vi "LinearSystemId_CreateDriveTrainSystem.vi"(4 "G":dbl, 6 "JKgMetersSquared":dbl, 8 "rbMeters":dbl, 9 "rMeters":dbl, 10 "MassKg":dbl, 11 "Motor":T1 {"Kt_NMPerAmp" format="%13.5p"; "Kv_RadPerSecPerVolt" format="%13.5p"; "R_Ohms" format="%13.5p"; "FreeSpeed_RadPerSec" format="%13.5p"; "FreeCurrent_Amps" format="%13.5p"; "StallCurrent_Amps" format="%13.5p"; "StallTorque_NM" format="%13.5p"; "nominalVoltage_Volts" format="%13.5p"}) -> (3 "Linearsystem":T2)   [LabVIEW 2019, in "Trajectory_Library.lvlib"]
doc: "Creates a new LINEAR SYSTEM data cluster with the specified values. \n\n\nInputs: \n - XXX -- XXX.\n\nOutputs:\n - XXX -- XXX."
uses:
  Trajectory_Library.lvlib
  LINEAR_SYSTEM.ctl
  <vilib>/Analysis/Matrix/Datatypes/RealMatrix.ctl
  DCMOTOR.CTL
  <vilib>/Analysis/Matrix/NI_Matrix.lvlib
panel:
  in  "Outputs":i32=2
  in  "Inputs":i32=2
  in  "States":i32=2
  # "<States,States>"
  # "<States,Inputs>"
  # "<Outputs,States>"
  # "<Outputs,Inputs>"
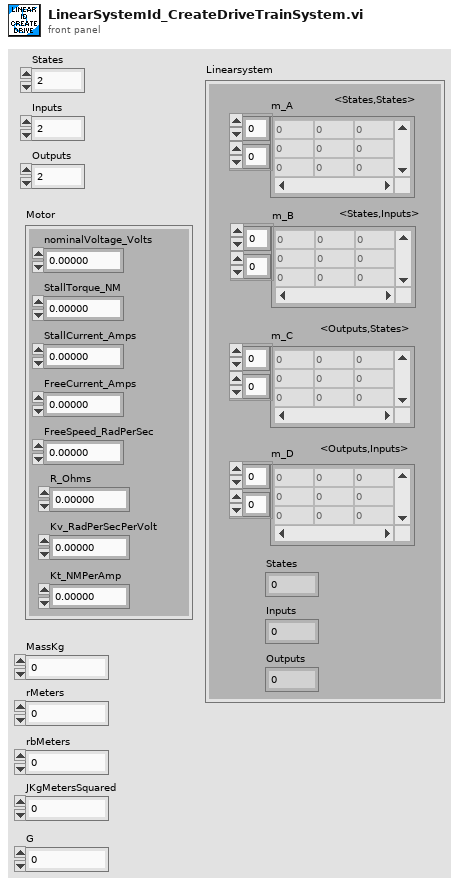
[diagram p1: front panel]
types:
  T1 = typedef "Trajectory_Library.lvlib/DCMOTOR.CTL" = cluster{"nominalVoltage_Volts":dbl, "StallTorque_NM":dbl, "StallCurrent_Amps":dbl, "FreeCurrent_Amps":dbl, "FreeSpeed_RadPerSec":dbl, "R_Ohms":dbl, "Kv_RadPerSecPerVolt":dbl, "Kt_NMPerAmp":dbl}
  T2 = typedef "Trajectory_Library.lvlib/LINEAR_SYSTEM.ctl" = cluster{"m_A":T3, "m_B":T3, "m_C":T3, "m_D":T3, "States":i32, "Inputs":i32, "Outputs":i32}
  T3 = typedef "NI_Matrix.lvlib/RealMatrix.ctl" = dbl[][]
  T4 = typedef "Trajectory_Library.lvlib/LINEARSYSTEM.ctl" = cluster{"m_A":T3, "m_B":T3, "m_C":T3, "m_D":T3, "States":i32, "Inputs":i32, "Outputs":i32}
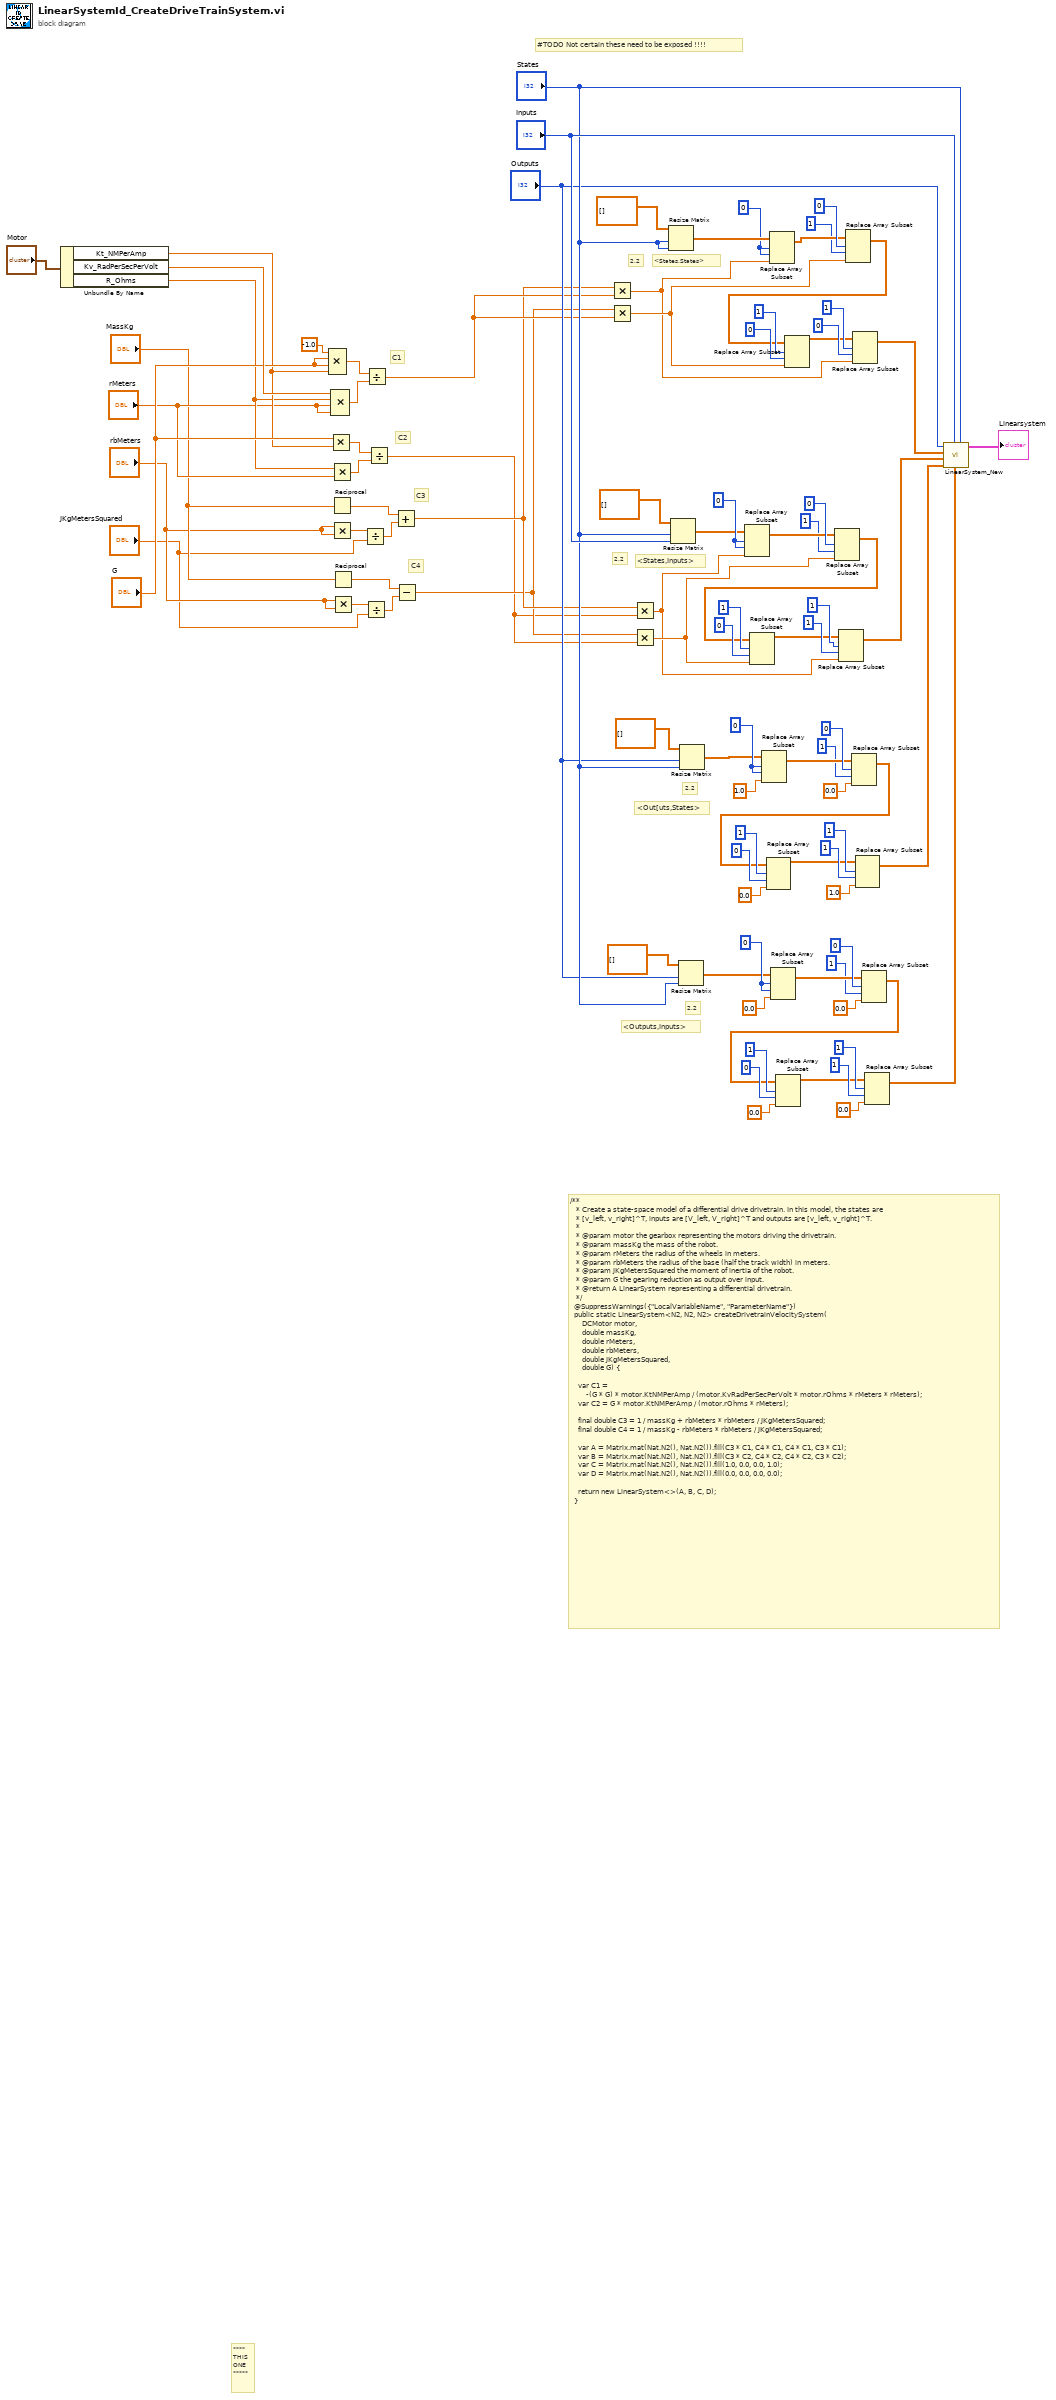
[diagram p0: block diagram]
diagram:
  w40 = 0 ("index (col)")
  w56 = 0 ("index (col)")
  w86 = 0 ("index (col)")
  w89 = 0 ("index (col)")
  # "C4"
  # "C3"
  # "C2"
  # "C1"
  # "2,2"
  # "2,2"
  # "2,2"
  # "2,2"
  # "<States,States>"
  # "<States,Inputs>"
  # "<Out[uts,States>"
  # "<Outputs,Inputs>"
  # "#TODO Not certain these need to be exposed !!!!"
  # "/**\n   * Create a state-space model of a differential drive drivetrain. In this model, the states are\n   * [v_left, v_right]^T, inputs are [V_left, V_right]^T and outputs are [v_left, v_right]^T.\n   *\n   * @param motor the gearbox representing the motors driving the drivetrain.\n   * @param massKg the mass of the robot.\n   * @param rMeters the radius of the wheels in meters.\n   * @param rbMeters the radius of the base (half the track width) in meters.\n   * @param JKgMetersSquared the moment of inertia of the robot.\n   * @param G the gearing reduction as output over input.\n   * @return A LinearSystem representing a differential drivetrain.\n   */\n  @SuppressWarnings({\"LocalVariableName\", \"ParameterName\"})\n  public static LinearSystem<N2, N2, N2> createDrivetrainVelocitySystem(\n      DCMotor motor,\n      double massKg,\n      double rMeters,\n      double rbMeters,\n      double JKgMetersSquared,\n      double G) {\n\n    var C1 =\n        -(G * G) * motor.KtNMPerAmp / (motor.KvRadPerSecPerVolt * motor.rOhms * rMeters * rMeters);\n    var C2 = G * motor.KtNMPerAmp / (motor.rOhms * rMeters);\n\n    final double C3 = 1 / massKg + rbMeters * rbMeters / JKgMetersSquared;\n    final double C4 = 1 / massKg - rbMeters * rbMeters / JKgMetersSquared;\n\n    var A = Matrix.mat(Nat.N2(), Nat.N2()).fill(C3 * C1, C4 * C1, C4 * C1, C3 * C1);\n    var B = Matrix.mat(Nat.N2(), Nat.N2()).fill(C3 * C2, C4 * C2, C4 * C2, C3 * C2);\n    var C = Matrix.mat(Nat.N2(), Nat.N2()).fill(1.0, 0.0, 0.0, 1.0);\n    var D = Matrix.mat(Nat.N2(), Nat.N2()).fill(0.0, 0.0, 0.0, 0.0);\n\n    return new LinearSystem<>(A, B, C, D);\n  }"
  # "****\nTHIS\nONE\n*****"
  n1 = Unbundle By Name("Motor") -> ("Kt_NMPerAmp"=w22:dbl, "Kv_RadPerSecPerVolt"=w26:dbl, "R_Ohms"=w19:dbl)
  n2 = Compound Arithmetic op=MULTIPLY(-1.0 ("value"), "G", "G", w22) -> (w25:dbl)
  n3 = Multiply(x="G", y=w22) -> (x*y=w21:dbl)
  n4 = Multiply(x=w19, y="rMeters") -> (x*y=w20:dbl)
  n5 = Reciprocal(x="MassKg") -> (1/x=w16:dbl)
  n6 = Multiply(x="rbMeters", y="rbMeters") -> (x*y=w17:dbl)
  n7 = Compound Arithmetic op=MULTIPLY(w26, w19, "rMeters", "rMeters") -> (w24:dbl)
  n8 = Reciprocal(x="MassKg") -> (1/x=w13:dbl)
  n9 = Multiply(x="rbMeters", y="rbMeters") -> (x*y=w14:dbl)
  n10 = Divide(x=w17, y="JKgMetersSquared") -> (x/y=w15:dbl)
  n11 = Divide(x=w14, y="JKgMetersSquared") -> (x/y=w12:dbl)
  n12 = Divide(x=w25, y=w24) -> (x/y=w8:dbl)
  n13 = Divide(x=w21, y=w20) -> (x/y=w3:dbl)
  n14 = Add(x=w16, y=w15) -> (x+y=w5:dbl)
  n15 = Subtract(x=w13, y=w12) -> (x-y=w4:dbl)
  n16 = Multiply(x=w5, y=w8) -> (x*y=w6:dbl)
  n17 = Multiply(x=w4, y=w8) -> (x*y=w7:dbl)
  n18 = Multiply(x=w5, y=w3) -> (x*y=w1:dbl)
  n19 = Multiply(x=w4, y=w3) -> (x*y=w2:dbl)
  n20 = Resize Matrix(1:"States", 2:"States", 4:T3 [] ("matrix")) -> (0:w90:T3)
  n21 = Resize Matrix(1:"Inputs", 2:"States", 4:T3 [] ("matrix")) -> (0:w33:T3)
  n22 = Resize Matrix(1:"States", 2:"Outputs", 4:T3 [] ("matrix")) -> (0:w42:T3)
  n23 = Resize Matrix(1:"States", 2:"Outputs", 4:T3 [] ("matrix")) -> (0:w84:T3)
  n24 = Replace Array Subset(array=w33, new element=w1, index (row)=w40, index (col)=w40) -> (w38:T3)
  n25 = Replace Array Subset(array=w84, new element=1.0 ("new element/submatrix"), index (row)=w86, index (col)=w86) -> (w83:T3)
  n26 = Replace Array Subset(array=w90, new element=w6, index (row)=w89, index (col)=w89) -> (w74:T3)
  n27 = Replace Array Subset(array=w42, new element=0.0 ("new element/submatrix"), index (row)=w56, index (col)=w56) -> (w54:T3)
  n28 = Replace Array Subset(array=w38, new element=w2, index (row)=0 ("index (col)"), index (col)=1 ("disabled index (col)")) -> (w32:T3)
  n29 = Replace Array Subset(array=w32, new element=w2, index (row)=1 ("index (col)"), index (col)=0 ("disabled index (col)")) -> (w30:T3)
  n30 = Replace Array Subset(array=w30, new element=w1, index (row)=1 ("index (col)"), index (col)=1 ("disabled index (col)")) -> (w29:T3)
  n31 = Replace Array Subset(array=w74, new element=w7, index (row)=0 ("index (col)"), index (col)=1 ("disabled index (col)")) -> (w67:T3)
  n32 = Replace Array Subset(array=w67, new element=w7, index (row)=1 ("index (col)"), index (col)=0 ("disabled index (col)")) -> (w68:T3)
  n33 = Replace Array Subset(array=w83, new element=0.0 ("new element/submatrix"), index (row)=0 ("index (col)"), index (col)=1 ("disabled index (col)")) -> (w59:T3)
  n34 = Replace Array Subset(array=w59, new element=0.0 ("new element/submatrix"), index (row)=1 ("index (col)"), index (col)=0 ("disabled index (col)")) -> (w57:T3)
  n35 = Replace Array Subset(array=w68, new element=w6, index (row)=1 ("index (col)"), index (col)=0 ("disabled index (col)")) -> (w66:T3)
  n36 = Replace Array Subset(array=w57, new element=1.0 ("new element/submatrix"), index (row)=1 ("index (col)"), index (col)=1 ("disabled index (col)")) -> (w58:T3)
  n37 = Replace Array Subset(array=w54, new element=0.0 ("new element/submatrix"), index (row)=0 ("index (col)"), index (col)=1 ("disabled index (col)")) -> (w44:T3)
  n38 = Replace Array Subset(array=w44, new element=0.0 ("new element/submatrix"), index (row)=1 ("index (col)"), index (col)=0 ("disabled index (col)")) -> (w43:T3)
  n39 = Replace Array Subset(array=w43, new element=0.0 ("new element/submatrix"), index (row)=1 ("index (col)"), index (col)=1 ("disabled index (col)")) -> (w41:T3)
  n40 = call "LinearSystem_New.vi"("States"="States", "D"=w41, "Inputs"="Inputs", "C"=w58, "B"=w29, "A"=w66, "Outputs"="Outputs") -> ("Linearsystem"=→"Linearsystem":T4)  [unwired: 4 in]
